vi "TEST VISA - Write CMD.vi"(6 "Index":i32, 8 "error in":errorcluster, 9 "Data":T1={"Test"={"Target Load"=0.0, "Target Disp"=0.0, "Rate"=0.0, "Speed"=0.0}, "Sensor"={"Name"=[], "Unit"=[], "Decimal Point"=[], "Ch Log"=[], "H Alarm"=[], "L Alarm"=[], "H Limit"=[], "L Limit"=[], "Filter"=[], "Gain"=[], "Calib Type"=[]}, "PID"={"SP"=0.0, "PV"=0.0, "kP"=0.0, "kI"=0.0, "kD"=0.0, "FF"=0.0, "Err Band"=0.0, "Max"=0, "Min"=0, "Ts"=0, "Out"=0, "Mode"=0}, "ADC"={"Active Ch"=[], "Filter Type"=0, "Post Filter"=[], "Gain"=[], "FS"=0, "IntOC"=0, "IntFC"=0, "SysOC"=0, "Cofficient"=[], "K"=[], "Max"=0}, "System"={"Out Type"=0, "Inverse"=0, "Monitor"=0, "Reserve"=0, "ACC Time"=0, "Pulse Rev"=0, "Stroke"=0, "Auto Off"=0, "Gear Ratio"=0.0, "Pitch"=0.0, "Max Speed"=0, "Jog Speed"=0, "Disp Coff"=0.0, "Max Load"=0}, "Index"=enum."Ch1", "Datalog"=enum."Empty"}, 10 "Action":T2) -> (0 "error out":errorcluster, 1 "Data Unit":T3, 2 "Data Channel":T4, 3 "VISA ref out":refnum<visa-resource-name>, 4 "Success":bool, 5 "Bytes at Port":u32, 7 "Prev Data?":bool)   [LabVIEW 2019]
uses:
  Controls/UDP - Command.ctl
  Controls/Communication - Write Data.ctl
  <vilib>/Instr/_visa.llb/VISA Flush IO Buffer Mask.ctl
  <vilib>/Instr/_visa.llb/VISA Configure Serial Port (Instr).vi
  Controls/Global - IP Address.vi
  Controls/Global - Handle V1.vi
  Controls/eFGV States.ctl
panel:
  out "read buffer":string
  out "error Parse Flush":errorcluster
  out "error parse":errorcluster
  out "error read":errorcluster
  out "error Write":errorcluster
  out "error Open Flush":errorcluster
  out "error open connection":errorcluster
  in  "Enable Termination\nChar (T)":bool=TRUE
  in  "VISA resource name":refnum<visa-resource-name>="COM6"
  out "x+y":i32
  out "error out 2":errorcluster
  out "appended array":u8[](array[numeric])
  out "*(type *) &x":string
  out "Raw Result":u8[](array[numeric])
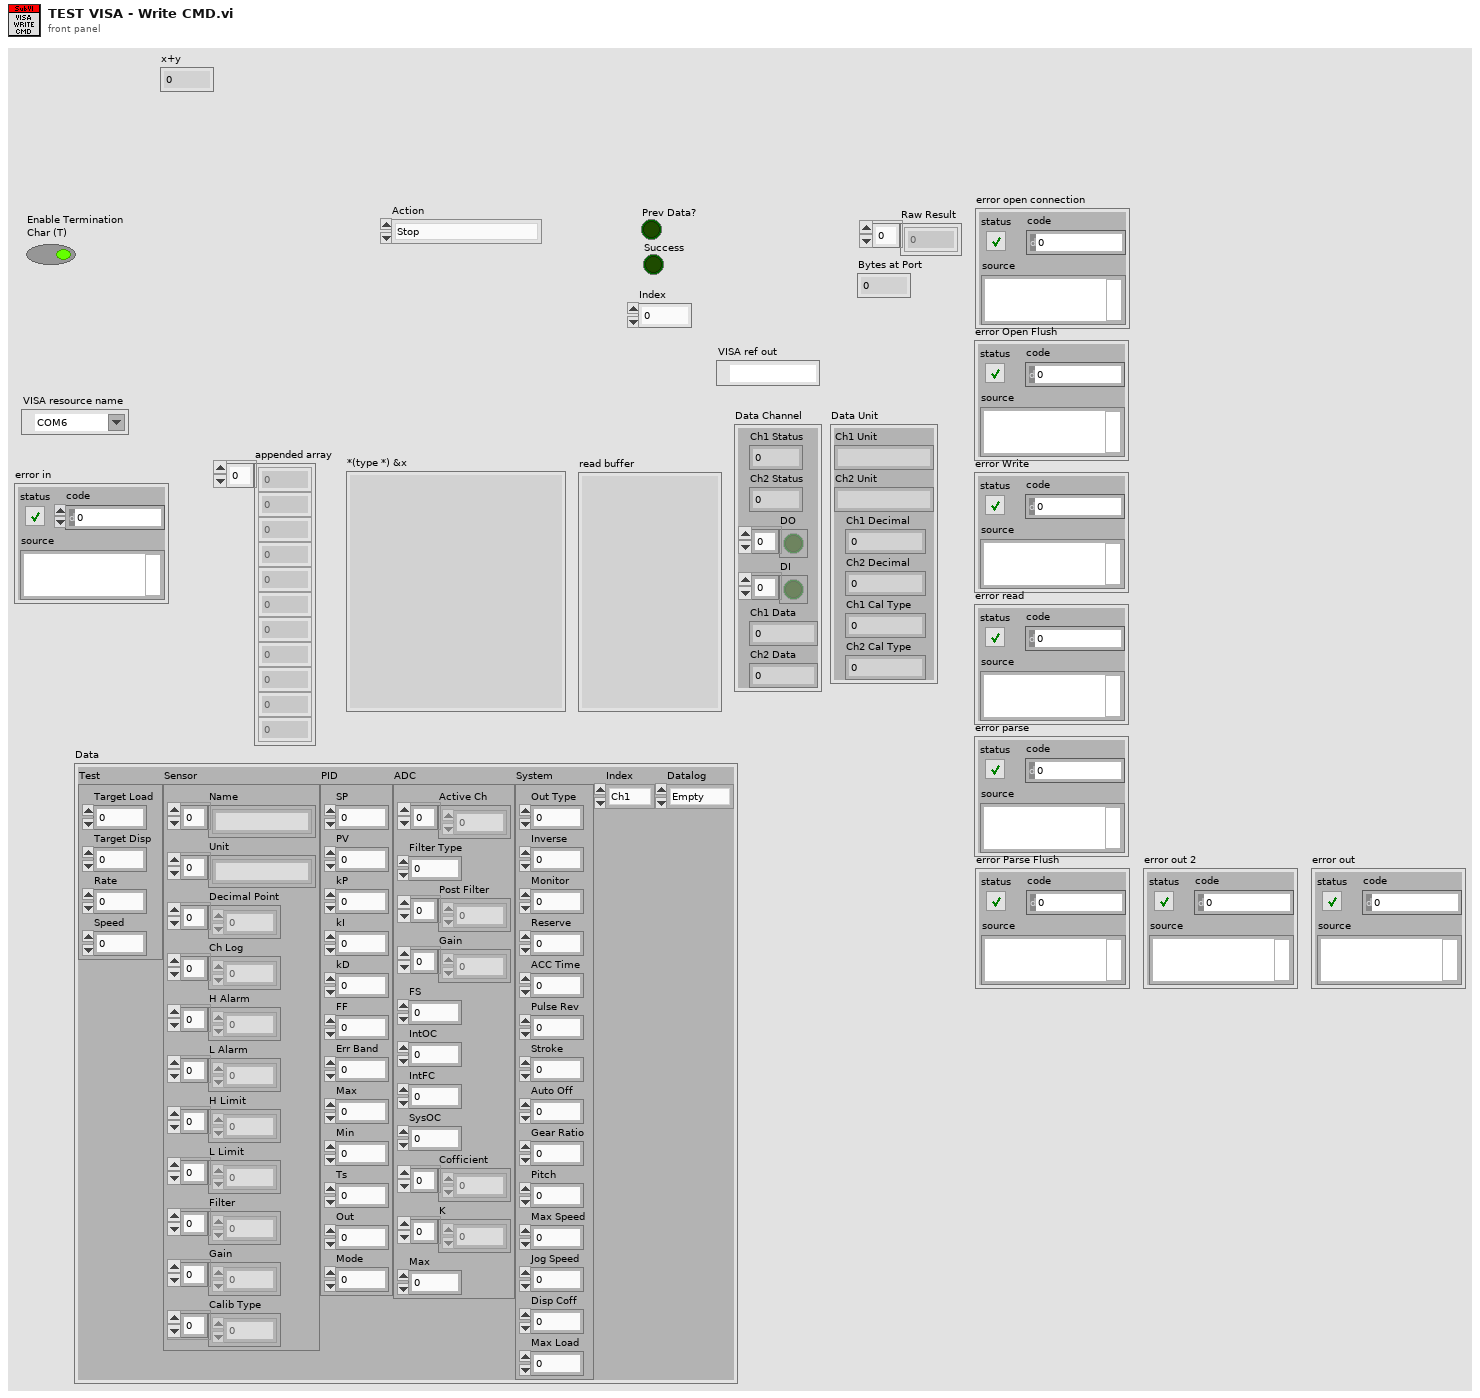
[diagram p1: front panel]
types:
  T1 = typedef "Communication - Write Data.ctl" = cluster{"Test":cluster{"Target Load":sgl, "Target Disp":sgl, "Rate":sgl, "Speed":sgl}, "Sensor":cluster{"Name":string[], "Unit":string[], "Decimal Point":u8[], "Ch Log":u8[], "H Alarm":u8[], "L Alarm":u8[], "H Limit":sgl[], "L Limit":sgl[], "Filter":u8[], "Gain":u8[], "Calib Type":u32[]}, "PID":cluster{"SP":sgl, "PV":sgl, "kP":sgl, "kI":sgl, "kD":sgl, "FF":sgl, "Err Band":sgl, "Max":i32, "Min":i32, "Ts":u32, "Out":i32, "Mode":u8}, "ADC":cluster{"Active Ch":u8[], "Filter Type":u8, "Post Filter":u8[], "Gain":u8[], "FS":u16, "IntOC":u8, "IntFC":u8, "SysOC":u8, "Cofficient":dbl[], "K":dbl[], "Max":i32}, "System":cluster{"Out Type":u8, "Inverse":u8, "Monitor":u8, "Reserve":u8, "ACC Time":u32, "Pulse Rev":u32, "Stroke":u32, "Auto Off":u32, "Gear Ratio":sgl, "Pitch":sgl, "Max Speed":u32, "Jog Speed":u32, "Disp Coff":sgl, "Max Load":u32}, "Index":enum16{"Ch1", "Ch2", "Ch3", "Ch4", "Ch5", "Ch6", "Ch7", "Ch8", "Ch9", "Ch10", "Ch11", "Ch12", "Ch13", "Ch14", "Ch15", "Ch16"}, "Datalog":enum16{"Ch1-Ch16", "Ch17-Ch32", "Ch32-Ch48", "Ch49-Ch64", "Empty"}}
  T2 = typedef "UDP - Command.ctl" = enum16{"Stop", "Jog Up", "Jog Down", "Ramp Up", "Ramp Down", "PID Target", "PID Ramp", "Disp Run", "Read Ch Data", "Zero Channel", "Zero Disp", "Read Sensor", "Write Sensor", "Read ADC", "Write ADC", "Read PID", "Write PID", "Read Test", "Write Test", "Read System", "Write System", "Read Datalog", "Read Datalog Sensor"}
  T3 = cluster{"Ch1 Unit":string, "Ch2 Unit":string, "Ch1 Decimal":u8, "Ch2 Decimal":u8, "Ch1 Cal Type":u8, "Ch2 Cal Type":u8}
  T4 = cluster{"Ch1 Status":u8, "Ch2 Status":u8, "DO":bool[], "DI":bool[], "Ch1 Data":sgl, "Ch2 Data":sgl}
  T5 = typedef "VISA Flush IO Buffer Mask.ctl" = u16
  T6 = typedef "eFGV States.ctl" = enum16{"Init", "Read", "Write", "Exit"}
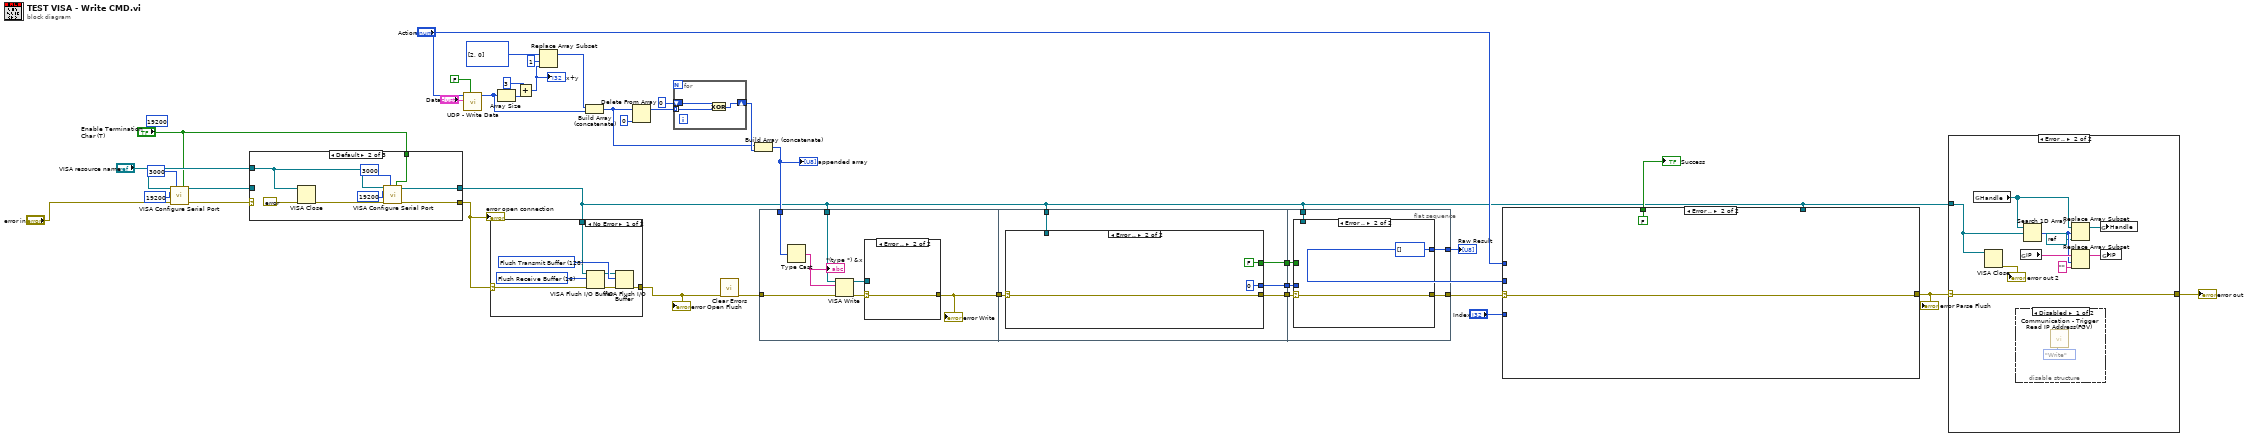
[diagram p0: block diagram]
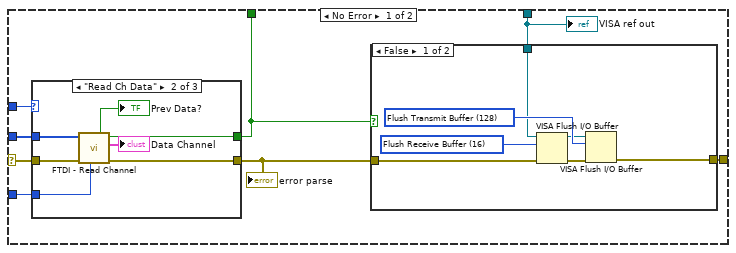
[diagram p2: hidden frame]
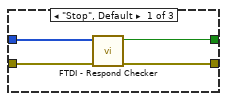
[diagram p4: hidden frame]
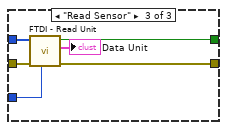
[diagram p5: hidden frame]
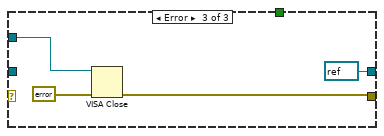
[diagram p8: hidden frame]
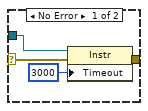
[diagram p11: hidden frame]
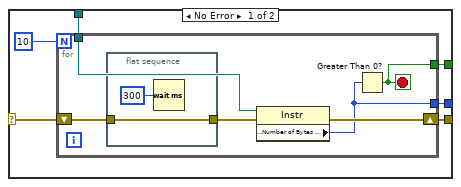
[diagram p12: hidden frame]
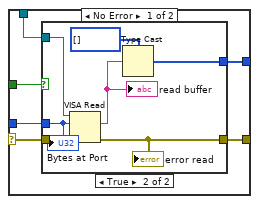
[diagram p13: hidden frame]
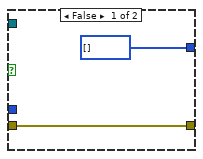
[diagram p14: hidden frame]
diagram:
  (unwired) u32 19200 ("baud rate (9600)")
  n1 = call-poly "VISA Configure Serial Port"("VISA resource name"="VISA resource name", "timeout (10sec)"=u32 3000, "Enable Termination\nChar (T)"="Enable Termination\nChar (T)", "baud rate (9600)"=u32 19200, "error in (no error)"="error in") -> ("VISA resource name out"=w10:refnum<visa-resource-name>, "error out"=w11:errorcluster)  [unwired: 9 in]
  n2 = case shown="Default" w11 {
    selector: w11 -> [w38 _ _]
    tunnel: [w39 w43 refnum<visa-resource-name> refnum ("VISA resource name out")] -> w2
    tunnel: w10 -> [w39 _ _]
    tunnel: [w38 w42 w49] -> w7
    tunnel: "VISA resource name" -> [_ w44 w50]
    tunnel: "Enable Termination\nChar (T)" -> [_ w40 _]
    frame No Error {
    }
    frame Default {
      n3 = VISA Close(VISA resource name=w44, error in (no error)=errorcluster {"status"=FALSE, "code"=0, "source"=""} ("error IO")) -> (error out=w45:errorcluster)
      n4 = call-poly "VISA Configure Serial Port"("VISA resource name"=w44, "timeout (10sec)"=u32 3000, "Enable Termination\nChar (T)"=w40, "baud rate (9600)"=u32 19200, "error in (no error)"=w45) -> ("VISA resource name out"=w43:refnum<visa-resource-name>, "error out"=w42:errorcluster)  [unwired: 9 in]
    }
    frame Error {
      n5 = VISA Close(VISA resource name=w50, error in (no error)=errorcluster {"status"=FALSE, "code"=0, "source"=""} ("error IO")) -> (error out=w49:errorcluster)
    }
  }
  "error open connection" <- w7
  n6 = call "UDP - Write Data.vi"("V2"=FALSE, "Data"="Data", "CMD"="Action") -> ("Array"=w25:u8[])  [unwired: 8 in]
  n7 = case shown="No Error" w7 {
    selector: w7 -> [w52 w59]
    tunnel: [w54 w59] -> w6
    tunnel: w2 -> [w53 _]
    frame No Error {
      w57 = T5 128 items=["Flush Receive Buffer"=16, "Write Transmit Buffer to Device"=32, "Flush Receive Buffer (No I/O)"=64, "Flush Transmit Buffer"=128] ("Mask")
      w58 = T5 16 items=["Flush Receive Buffer"=16, "Write Transmit Buffer to Device"=32, "Flush Receive Buffer (No I/O)"=64, "Flush Transmit Buffer"=128] ("Mask")
      n8 = VISA Flush I/O Buffer(VISA resource name=w53, mask (16)=w58, error in (no error)=w52) -> (VISA resource name out=w55:refnum<visa-resource-name>, error out=w56:errorcluster)
      n9 = VISA Flush I/O Buffer(VISA resource name=w55, mask (16)=w57, error in (no error)=w56) -> (error out=w54:errorcluster)  [unwired: 1 out]
    }
    frame Error {
    }
  }
  "error Open Flush" <- w6
  n10 = Array Size(array=w25) -> (size(s)=w21:i32)
  n11 = Add(x=3, y=w21) -> (x+y=w19:i32)
  "x+y" <- w19
  n12 = Replace Array Subset(array=u8[] [2, 0], new element=w19, index=1) -> (w22:u8[])
  n13 = Build Array (concatenate)(w22, w25) -> (w16:u8[])
  n14 = Delete From Array(array=w16, index=0) -> (array with subset deleted=w35:u8[])  [unwired: 1 in, 1 out]
  n15 = for {
    shift-right: [w61] -> w34
    shift-left: u8 0 ("Numeric") -> [w62]
    tunnel: w35 -> [w60] mode=indexing
    n16 = Exclusive Or(1:w60, 2:w62) -> (0:w61:u8)
  }
  n17 = call <vilib>:"Clear Errors.vi"("error in (no error)"=w6) -> ("error out"=w4:errorcluster)  [unwired: 5 in, 1 out]
  n18 = Build Array (concatenate)(w16, w34) -> (w33:u8[])
  "appended array" <- w33
  n19 = flat-sequence {
    tunnel: w33 -> [w67]
    tunnel: [w65] -> w28
    tunnel: w2 -> [w68]
    tunnel: w4 -> [w69]
    tunnel: [w79] -> w32
    tunnel: w28 -> [w75]
    tunnel: w2 -> [w78]
    tunnel: [w77] -> w30
    tunnel: [w76] -> w13
    tunnel: [w100] -> w31
    tunnel: [w102] -> w1
    tunnel: w32 -> [w97]
    tunnel: w2 -> [w101]
    tunnel: w30 -> [w99]
    tunnel: w13 -> [w98]
    frame #0 {
      n20 = Type Cast(x=w67) -> (*(type *) &x=w66:string)  [unwired: 1 in]
      "*(type *) &x" <- w66
      n21 = VISA Write(VISA resource name=w68, write buffer=w66, error in (no error)=w69) -> (VISA resource name out=w64:refnum<visa-resource-name>, error out=w63:errorcluster)  [unwired: 1 out]
      n22 = case shown="Error .." w63 {
        selector: w63 -> [w70 w74]
        tunnel: [w73 w74] -> w65
        tunnel: w64 -> [w72 _]
        frame No Error {
          n23 = property class="Instr"(reference=w72, error in=w70, "Timeout"=u32 3000 ("General Settings:Timeout Value")) -> (error out=w73:errorcluster)  [unwired: 1 out]
        }
        frame Error {
        }
      }
      "error Write" <- w65
    }
    frame #1 {
      n24 = case shown="Error .." w75 {
        selector: w75 -> [w80 w96]
        tunnel: [w85 w96] -> w79
        tunnel: w78 -> [w84 _]
        tunnel: [w83 u32 0 ("Bytes at Port")] -> w77
        tunnel: [w81 FALSE] -> w76
        frame No Error {
          n25 = for {
            N: 10 -> [_]
            tunnel: w84 -> [w90]
            tunnel: [w88] -> w83
            shift-right: [w91] -> w85
            shift-left: w80 -> [w86]
            tunnel: [w89] -> w81
            stop <- w89 stop-if-true
            n26 = flat-sequence {
              tunnel: [w92] -> w87
              tunnel: w86 -> [w92]
              frame #0 {
                n27 = Wait (ms)(milliseconds to wait=u32 300) -> ()  [unwired: 1 out]
              }
            }
            n28 = property class="Instr"(reference=w90, error in=w87) -> (error out=w91:errorcluster, "Serial Settings:Number of Bytes at Serial Port"=w88:u32)  [unwired: 1 out]
            n29 = Greater Than 0?(x=w88) -> (x > 0?=w89:bool)
          }
        }
        frame Error {
        }
      }
    }
    frame #2 {
      n30 = case shown="Error .." w97 {
        selector: w97 -> [w103 w118]
        tunnel: [w108 w118] -> w102
        tunnel: w101 -> [w107 _]
        tunnel: [w106 u8[] [] ("appended array")] -> w100
        tunnel: w99 -> [w105 _]
        tunnel: w98 -> [w104 _]
        frame No Error {
          n31 = case shown="True" w104 {
            tunnel: [w110 w117] -> w108
            tunnel: w103 -> [w110 w116]
            tunnel: w107 -> [_ w115]
            tunnel: w105 -> [_ w114]
            tunnel: [u8[] [] ("appended array") w111] -> w106
            frame False {
            }
            frame True {
              n32 = VISA Read(VISA resource name=w115, byte count=w114, error in (no error)=w116) -> (read buffer=w113:string, error out=w117:errorcluster)  [unwired: 2 out]
              "error read" <- w117
              "read buffer" <- w113
              n33 = Type Cast(type=u8[] [] ("appended array"), x=w113) -> (*(type *) &x=w111:u8[])
              "Bytes at Port" <- w114
            }
          }
        }
        frame Error {
        }
      }
    }
  }
  n34 = case shown="Error .." w1 {
    selector: w1 -> [w120 w153]
    tunnel: w31 -> [w127 _]
    tunnel: [w125 FALSE ("Success")] -> w29
    tunnel: [w124 w153] -> w27
    tunnel: "Action" -> [w123 _]
    tunnel: "Index" -> [w122 _]
    tunnel: w2 -> [w121 _]
    frame No Error {
      n35 = case shown="\"Read Ch Data\"" w123 {
        tunnel: [w138 w145 w148] -> w126
        tunnel: w120 -> [w138 w144 w151]
        tunnel: w127 -> [w137 w143 w150]
        tunnel: [w136 w142 w149] -> w125
        tunnel: w122 -> [_ w140 w146]
        frame "Stop", Default {
          n36 = call "FTDI - Respond Checker.vi"("Read Data"=w137) -> ("Success"=w136:bool)  [unwired: 10 in]
        }
        frame "Read Ch Data" {
          n37 = call "FTDI - Read Channel.vi"("index"=w140, "error in"=w144, "Result"=w143) -> ("error out"=w145:errorcluster, "Data Channel"=→"Data Channel":T4, "Success"=w142:bool, "Prev Data?"=→"Prev Data?":bool)  [unwired: 5 in]
        }
        frame "Read Sensor" {
          n38 = call "FTDI - Read Unit.vi"("Index"=w146, "error in"=w151, "Result"=w150) -> ("error out"=w148:errorcluster, "Data Unit"=→"Data Unit":T3, "Success"=w149:bool)  [unwired: 6 in]
        }
      }
      "error parse" <- w126
      n39 = case shown="False" w125 {
        tunnel: w126 -> [w130 w135]
        tunnel: [w128 w135] -> w124
        tunnel: w121 -> [w129 _]
        frame False {
          w133 = T5 128 items=["Flush Receive Buffer"=16, "Write Transmit Buffer to Device"=32, "Flush Receive Buffer (No I/O)"=64, "Flush Transmit Buffer"=128] ("Mask")
          w134 = T5 16 items=["Flush Receive Buffer"=16, "Write Transmit Buffer to Device"=32, "Flush Receive Buffer (No I/O)"=64, "Flush Transmit Buffer"=128] ("Mask")
          n40 = VISA Flush I/O Buffer(VISA resource name=w129, mask (16)=w134, error in (no error)=w130) -> (VISA resource name out=w131:refnum<visa-resource-name>, error out=w132:errorcluster)
          n41 = VISA Flush I/O Buffer(VISA resource name=w131, mask (16)=w133, error in (no error)=w132) -> (error out=w128:errorcluster)  [unwired: 1 out]
        }
        frame True {
        }
      }
      "VISA ref out" <- w121
    }
    frame Error {
    }
  }
  "Success" <- w29
  "error Parse Flush" <- w27
  n42 = case shown="Error .." w27 {
    selector: w27 -> [w154 w164]
    tunnel: [w154 w164] -> w26
    tunnel: w2 -> [_ w156]
    frame No Error {
    }
    frame Error {
      n43 = global read "Global - Handle V1.vi" "Handle"() -> (w163:refnum<visa-resource-name>[])
      n44 = VISA Close(VISA resource name=w156) -> (error out=→"error out 2":errorcluster)  [unwired: 1 in]
      n45 = disable-structure shown="Disabled" {
        frame Disabled {
          n46 = call "Communication - Trigger Read IP Address(FGV).vi"("Action"=eFGV_States."Write") -> ()  [unwired: 8 in, 3 out]
        }
        frame Enabled {
        }
      }
      n47 = global read "Global - IP Address.vi" "IP"() -> (w161:string[])
      n48 = Search 1D Array(1D array=w163, element=w156) -> (index of element=w160:i32)  [unwired: 1 in]
      n49 = Replace Array Subset(array=w163, new element=refnum<visa-resource-name> refnum ("new element/subarray"), index=w160) -> (w162:refnum<visa-resource-name>[])
      n50 = Replace Array Subset(array=w161, new element="" ("new element/subarray"), index=w160) -> (w159:string[])
      n51 = global write "Global - Handle V1.vi" "Handle"(w162) -> ()
      n52 = global write "Global - IP Address.vi" "IP"(w159) -> ()
    }
  }
  "error out" <- w26
  "Raw Result" <- w31
